vi "3D - A and B (SubVI).vi"(3 "Angle theta [degrees]":dbl, 4 "Total steps":dbl, 5 "Current step":dbl, 6 "Magnitude":dbl) -> (0 "B_B":dbl format="%#_6f", 1 "Current angle":dbl format="%#_6f", 2 "B_A":dbl format="%#_6f")   [LabVIEW 2018]
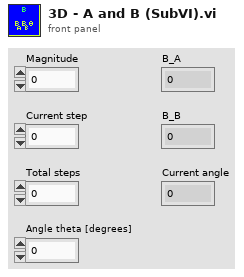
[diagram p1: front panel]
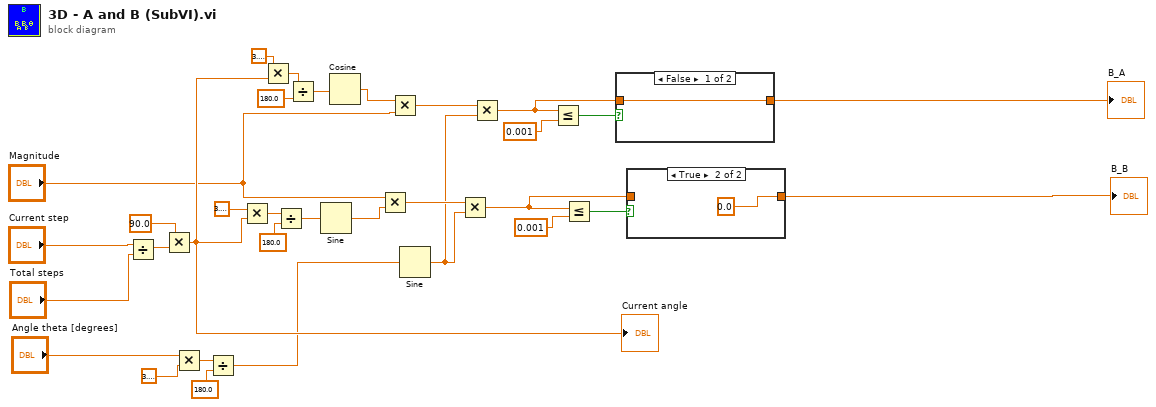
[diagram p0: block diagram]
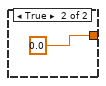
[diagram p3: hidden frame]
diagram:
  n1 = Divide(x="Current step", y="Total steps") -> (x/y=w30:dbl)
  n2 = Multiply(x=90.0, y=w30) -> (x*y=w32:dbl)
  "Current angle" <- w32
  n3 = Multiply(x="Angle theta [degrees]", y=3.141592653589793) -> (x*y=w14:dbl)
  n4 = Divide(x=w14, y=180.0) -> (x/y=w11:dbl)
  n5 = Multiply(x=3.141592653589793, y=w32) -> (x*y=w23:dbl)
  n6 = Multiply(x=3.141592653589793, y=w32) -> (x*y=w19:dbl)
  n7 = Divide(x=w23, y=180.0) -> (x/y=w22:dbl)
  n8 = Divide(x=w19, y=180.0) -> (x/y=w16:dbl)
  n9 = Sine(x=w22) -> (sin(x)=w25:dbl)
  n10 = Cosine(x=w16) -> (cos(x)=w24:dbl)
  n11 = Multiply(x="Magnitude", y=w25) -> (x*y=w27:dbl)
  n12 = Multiply(x=w24, y="Magnitude") -> (x*y=w26:dbl)
  n13 = Sine(x=w11) -> (sin(x)=w9:dbl)
  n14 = Multiply(x=w27, y=w9) -> (x*y=w3:dbl)
  n15 = Multiply(x=w26, y=w9) -> (x*y=w6:dbl)
  n16 = Less Or Equal?(x=w6, y=0.001) -> (x <= y?=w7:bool)
  n17 = Less Or Equal?(x=w3, y=0.001) -> (x <= y?=w4:bool)
  n18 = case shown="False" w7 {
    tunnel: [w33 0.0 ("y")] -> w2
    tunnel: w6 -> [w33 _]
    frame False {
    }
    frame True {
    }
  }
  "B_A" <- w2
  n19 = case shown="True" w4 {
    tunnel: [w35 0.0 ("y")] -> w1
    tunnel: w3 -> [w35 _]
    frame False {
    }
    frame True {
    }
  }
  "B_B" <- w1
